vi "mqttBuildUserInfo.vi"(0 "mqtt in":refnum<class "mqtt.lvclass">, 11 "error in (no error)":errorcluster) -> (4 "mqtt out":refnum<class "mqtt.lvclass">, 8 "userInfo out":u8[](array[numeric]), 15 "error out":errorcluster)   [LabVIEW 2022 SP3, in "mqtt.lvclass"]
uses:
  mqtt.lvclass
  mqtt.lvclass/mqtt.ctl
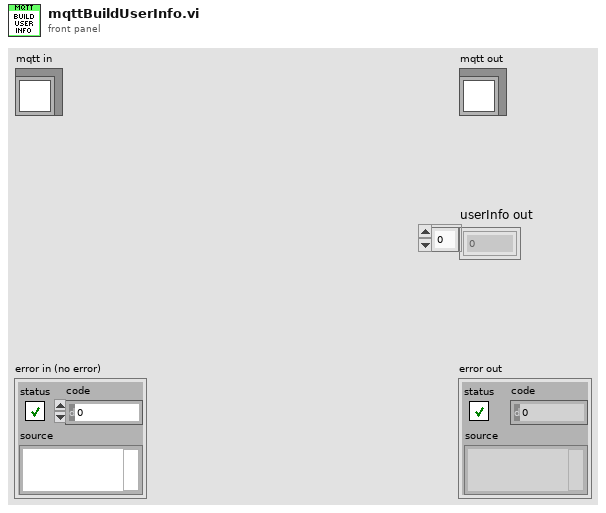
[diagram p1: front panel]
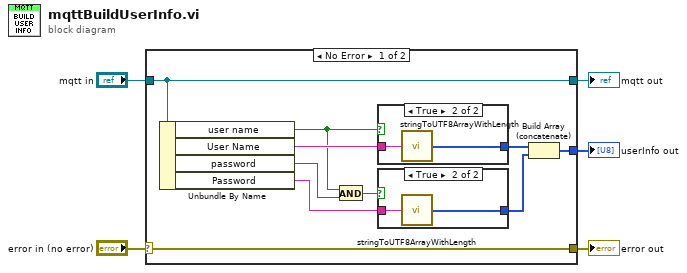
[diagram p0: block diagram]
diagram:
  n1 = case shown="No Error" "error in (no error)" {
    selector: "error in (no error)" -> [w15 w21]
    tunnel: [w15 w21] -> w4
    tunnel: [w14 w20] -> w2
    tunnel: "mqtt in" -> [w14 w20]
    tunnel: [w9 _] -> w1
    frame No Error {
      n2 = Unbundle By Name(w14) -> ("user name"=w7:bool, "User Name"=w12:string, "password"=w8:bool, "Password"=w13:string)
      n3 = And(x=w7, y=w8) -> (x .and. y?=w6:bool)
      n4 = case shown="True" w7 {
        tunnel: w12 -> [_ w17]
        tunnel: [_ w16] -> w11
        frame False {
        }
        frame True {
          n5 = call "stringToUTF8ArrayWithLength.vi"("string"=w17) -> ("UTF8[]"=w16:u8[])  [unwired: 14 in]
        }
      }
      n6 = case shown="True" w6 {
        tunnel: w13 -> [_ w19]
        tunnel: [_ w18] -> w10
        frame False {
        }
        frame True {
          n7 = call "stringToUTF8ArrayWithLength.vi"("string"=w19) -> ("UTF8[]"=w18:u8[])  [unwired: 14 in]
        }
      }
      n8 = Build Array (concatenate)(w11, w10) -> (w9:u8[])
    }
    frame Error {
    }
  }
  "error out" <- w4
  "mqtt out" <- w2
  "userInfo out" <- w1
